vi "timetest.vi"() -> ()   [LabVIEW 2015]
uses:
  BERTTA.dll
panel:
  in  "Delay Time (s)":dbl=1.0
  out "params":i32[](array[numeric])
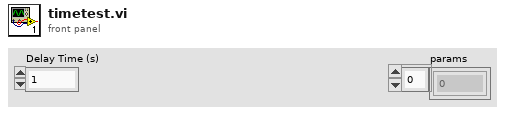
[diagram p1: front panel]
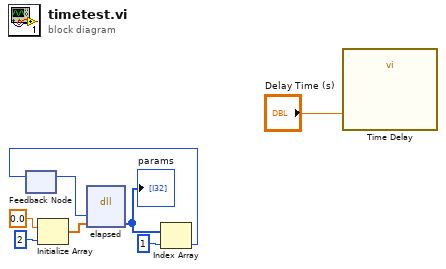
[diagram p0: block diagram]
diagram:
  n1 = feedback #1() -> (w6:i32)  [unwired: 1 in]
  n2 = Initialize Array(0.0 ("element"), 2 ("dimension size")) -> (w4:dbl[])
  n3 = dll-call lib="C:/Users/xlaraser/Documents/Visual Studio 2017/Projects/Bertta/BERTTA/Debug/BERTTA.dll" fn="elapsed"("last_time"=w6, "params"=w4) -> ("params"=w2:i32[])  [unwired: 5 in, 2 out]
  "params" <- w2
  n4 = Index Array(array=w2, index=1) -> (element=w7:i32)
  n5 = feedback-in #1(w7) -> ()
  n6 = call "Time Delay"("Delay Time (s)"="Delay Time (s)") -> ()  [unwired: 10 in, 1 out]
